vi "COVID_19_CSSE_JHU_Parser.vi"() -> ()   [LabVIEW 2015]
panel:
  out "Graph 2":cluster{"Array out":dbl[], "Array out":dbl[]}[](graph)
  out "Graph":cluster{"Array out":dbl[], dbl[]}[](graph)
  out "Preview":dbl[](graph)
  in  "Population (Millions)":u64 format="%.3p"
  in  "Adjusted by Population (Million)":bool
  in  "Align to First Cases Reported":bool
  in  "State/Province":string(combo)="All"
  in  "Country":string(combo)="All"
  in  "Dataset":enum32{"Confirmed Cases", "Deaths"}(radio)
  in  "Path":path
  in  "reset":bool
  in  "plot":bool
  in  "stop":bool
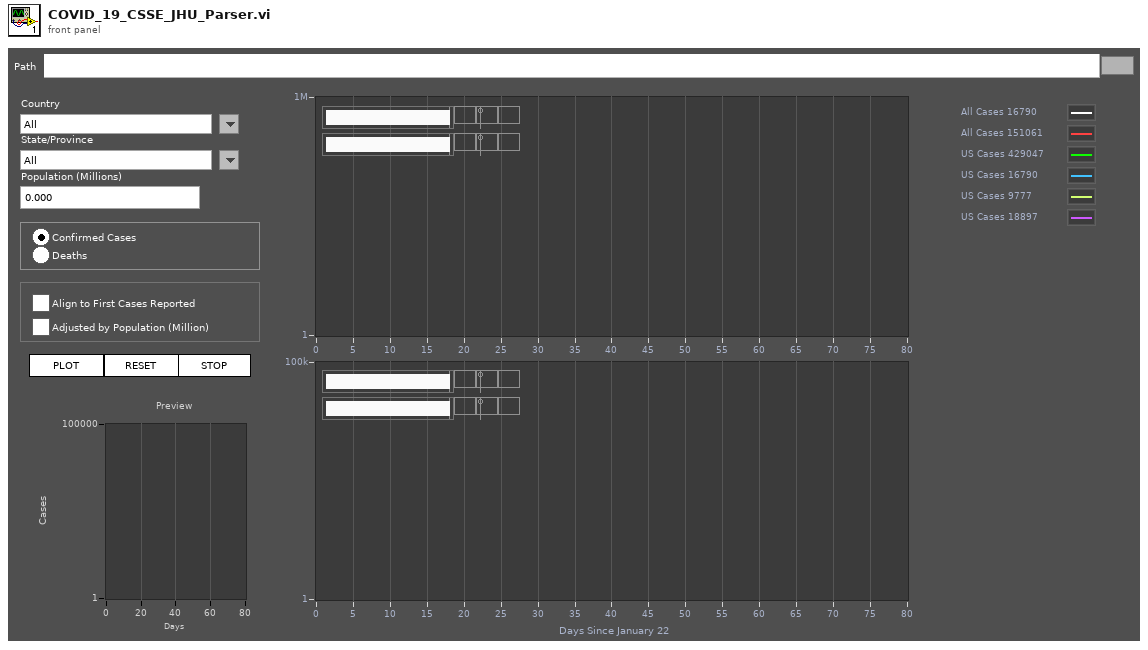
[diagram p1: front panel]
types:
  T1 = enum16{"Initialize", "Start", "Plot", "Reset", "Convert_Data"}
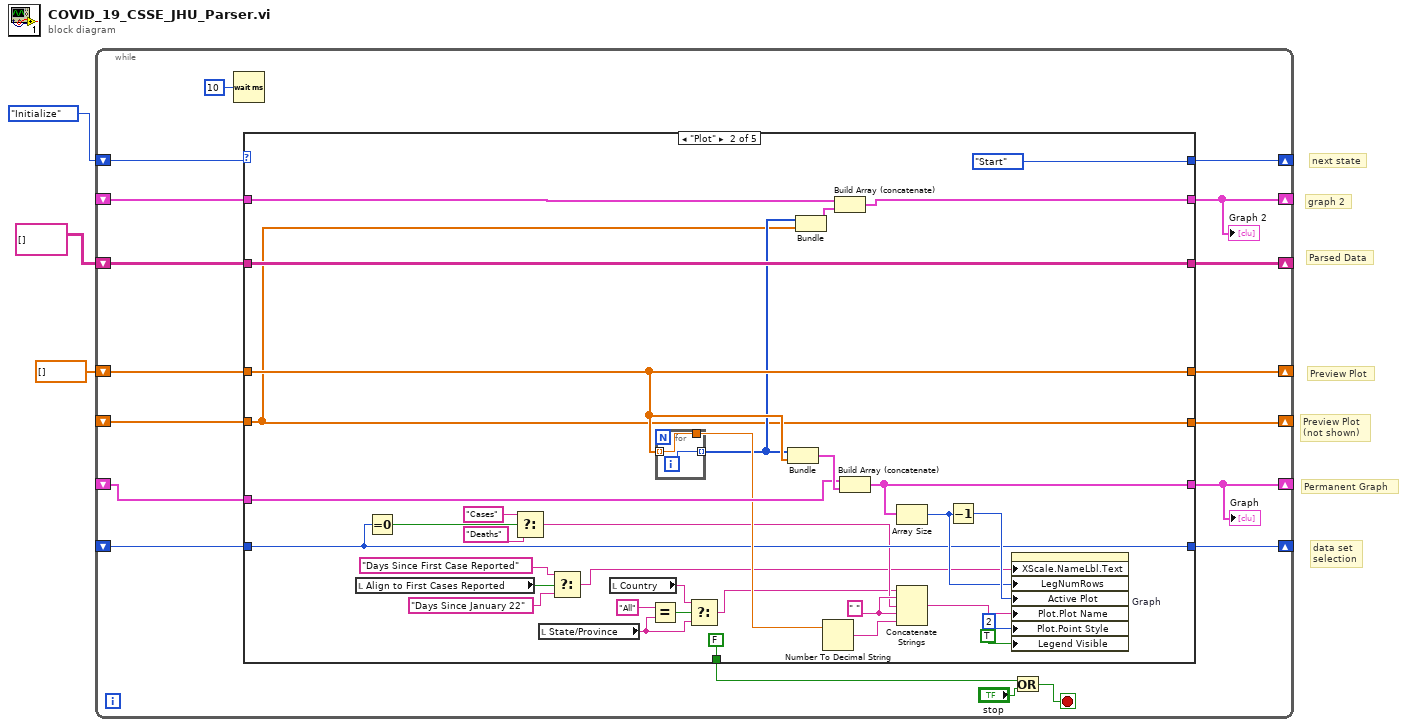
[diagram p0: block diagram]
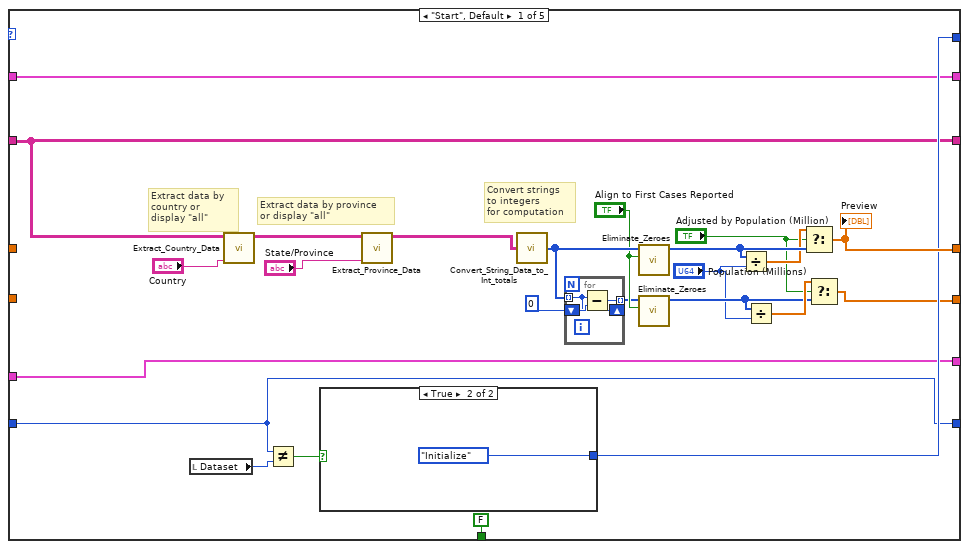
[diagram p2: hidden frame]
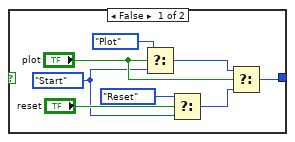
[diagram p3: hidden frame]
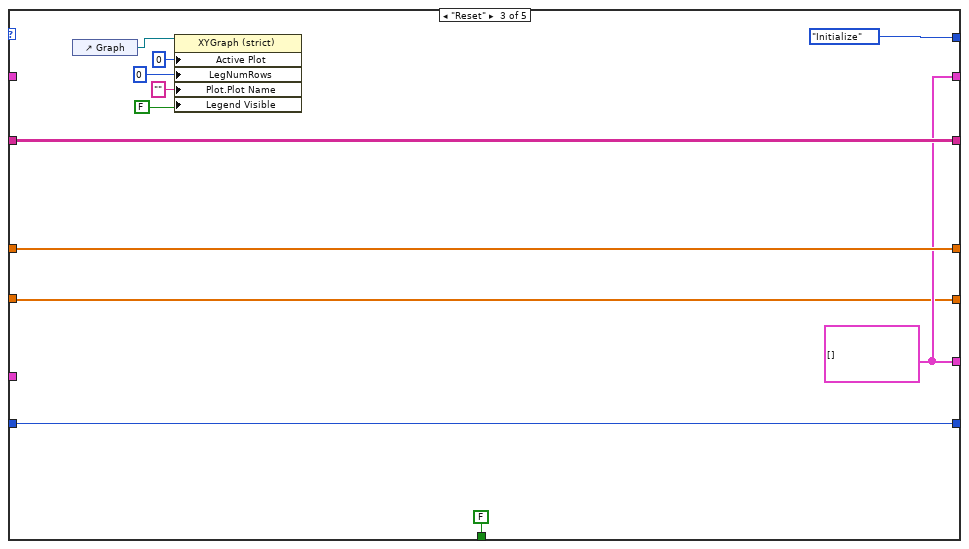
[diagram p4: hidden frame]
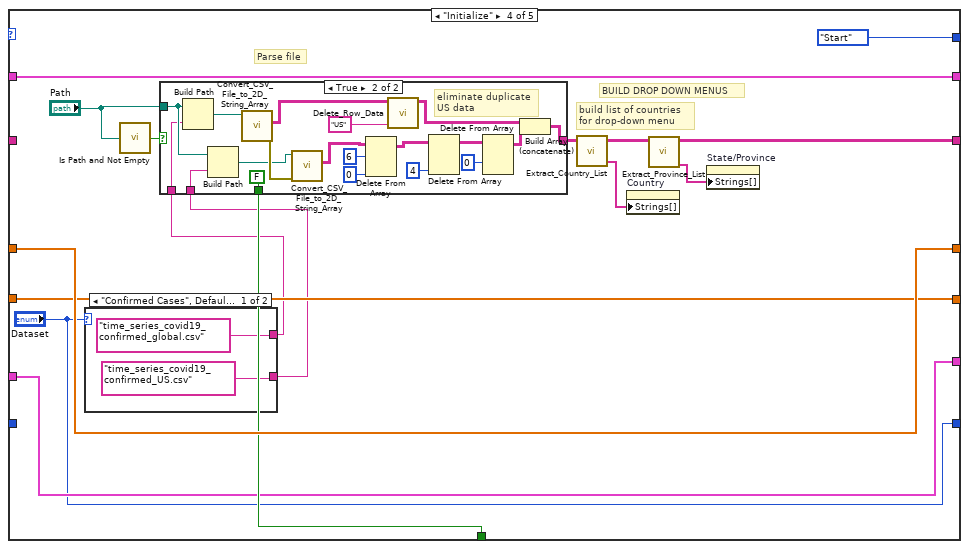
[diagram p5: hidden frame]
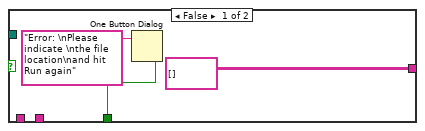
[diagram p6: hidden frame]
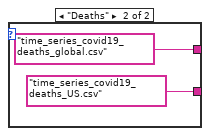
[diagram p7: hidden frame]
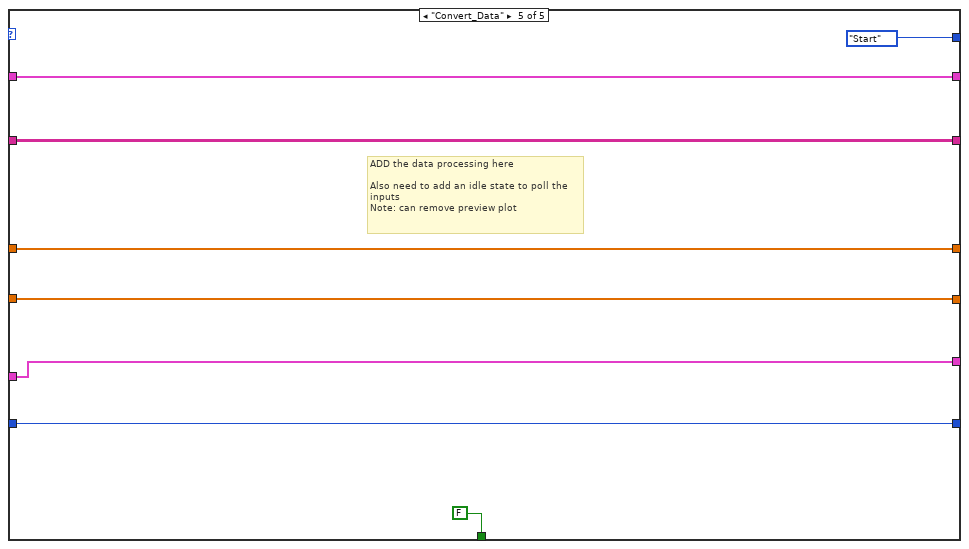
[diagram p8: hidden frame]
diagram:
  # "data set\nselection"
  # "next state"
  # "graph 2"
  # "Preview Plot \n(not shown)"
  # "Parsed Data"
  # "Preview Plot"
  # "Permanent Graph"
  n1 = while {
    shift-right: [w16] -> _
    shift-left: T1."Initialize" -> [w4]
    shift-right: [w20] -> _
    shift-left: string[][] [] ("all rows") -> [w19]
    shift-right: [w18] -> _
    shift-left: dbl[] [] ("Array out") -> [w17]
    shift-right: [w15] -> _
    shift-left: _ -> [w14]
    shift-right: [w13] -> _
    shift-left: _ -> [w12]
    shift-right: [w11] -> _
    shift-left: _ -> [w10]
    shift-right: [w8] -> _
    shift-left: _ -> [w9]
    stop <- w6 stop-if-true
    n2 = Wait (ms)(milliseconds to wait=u32 10) -> ()  [unwired: 1 out]
    n3 = case shown="\"Plot\"" w4 {
      tunnel: [w23 w91 w104 w108 w154] -> w20
      tunnel: w19 -> [w23 w91 w104 _ w154]
      tunnel: [w41 w87 w105 w121 w153] -> w18
      tunnel: w17 -> [_ w87 w105 w121 w153]
      tunnel: [w38 enum16{"Initialize", "Start", "Plot", "Reset"}."Start" enum16{"Initialize", "Start", "Plot", "Reset"}."Initialize" enum16{"Initialize", "Start", "Plot", "Reset"}."Start" T1."Start"] -> w16
      tunnel: [w37 w78 w102 "Dataset" w150] -> w15
      tunnel: w14 -> [w37 w78 w102 _ w150]
      tunnel: [w30 w86 w96 w114 w151] -> w13
      tunnel: w12 -> [w30 w88 _ w114 w151]
      tunnel: [w24 w64 w95 w119 w152] -> w11
      tunnel: w10 -> [_ w64 w95 w119 w152]
      tunnel: [w33 w66 w96 w118 w155] -> w8
      tunnel: w9 -> [w33 w65 _ w118 w155]
      tunnel: [FALSE ("true") FALSE ("true") FALSE ("true") w115 FALSE ("true")] -> w5
      frame "Start", Default {
        # "Extract data by province \nor display \"all\""
        # "Convert strings \nto integers\nfor computation"
        # "Extract data by country or display \"all\""
        n4 = local read "Dataset"() -> (w40:enum32{"Confirmed Cases", "Deaths"})
        n5 = call "Extract_Country_Data.vi"("Country"="Country", "Raw Data Array (String)"=w23) -> ("Country Data"=w22:string[][])  [unwired: 9 in]
        n6 = Not Equal?(x=w37, y=w40) -> (x != y?=w39:bool)
        n7 = case shown="True" w39 {
          tunnel: [w54 enum16{"Initialize", "Start", "Plot", "Reset"}."Initialize"] -> w38
          frame False {
            w50 = enum16{"Initialize", "Start", "Plot", "Reset"}."Start"
            n8 = Select(t=enum16{"Initialize", "Start", "Plot", "Reset"}."Plot", s="plot", f=w50) -> (s? t:f=w53:enum16{"Initialize", "Start", "Plot", "Reset"})
            n9 = Select(t=enum16{"Initialize", "Start", "Plot", "Reset"}."Reset", s="reset", f=w50) -> (s? t:f=w49:enum16{"Initialize", "Start", "Plot", "Reset"})
            n10 = Select(t=w53, s="plot", f=w49) -> (s? t:f=w54:enum16{"Initialize", "Start", "Plot", "Reset"})
          }
          frame True {
          }
        }
        n11 = call "Extract_Province_Data.vi"("Province"="State/Province", "Country Data In"=w22) -> ("Province Data Out"=w43:string[][])  [unwired: 9 in]
        n12 = call "Convert_String_Data_to_Int_totals.vi"("Province Data Out"=w43) -> ("Array"=w36:i32[])
        n13 = for {
          tunnel: w36 -> [w46] mode=indexing
          shift-right: [w46] -> _
          shift-left: 0 -> [w48]
          tunnel: [w47] -> w31 mode=indexing
          n14 = Subtract(x=w46, y=w48) -> (x-y=w47:i32)
        }
        n15 = call "Eliminate_Zeroes.vi"("Align to First Cases Reported"="Align to First Cases Reported", "Array in"=w36) -> ("Array out"=w42:i32[])  [unwired: 9 in]
        n16 = call "Eliminate_Zeroes.vi"("Align to First Cases Reported"="Align to First Cases Reported", "Array in"=w31) -> ("Array out"=w27:i32[])  [unwired: 9 in]
        n17 = Divide(x=w42, y="Population (Millions)") -> (x/y=w29:dbl[])
        n18 = Divide(x=w27, y="Population (Millions)") -> (x/y=w28:dbl[])
        n19 = Select(t=w29, s="Adjusted by Population (Million)", f=w42) -> (s? t:f=w41:dbl[])
        "Preview" <- w41
        n20 = Select(t=w28, s="Adjusted by Population (Million)", f=w27) -> (s? t:f=w24:dbl[])
      }
      frame "Plot" {
        w74 = " " ("string")
        n21 = local read "Align to First Cases Reported"() -> (w70:bool)
        n22 = Equal To 0?(x=w78) -> (x = 0?=w77:bool)
        n23 = Select(t="Cases" ("string"), s=w77, f="Deaths" ("string")) -> (s? t:f=w73:string)
        n24 = local read "State/Province"() -> (w59:string)
        n25 = Select(t="Days Since First Case Reported" ("string"), s=w70, f="Days Since January 22" ("string")) -> (s? t:f=w69:string)
        n26 = local read "Country"() -> (w60:string)
        n27 = Equal?(x="All", y=w59) -> (x = y?=w61:bool)
        n28 = for {
          tunnel: w87 -> [w93] mode=indexing
          tunnel: [w92] -> w67 mode=indexing
          tunnel: [w93] -> w79
          i -> [w92]
        }
        n29 = Select(t=w60, s=w61, f=w59) -> (s? t:f=w58:string)
        n30 = Bundle(w67, "Array out"=w87) -> (w89:cluster{i32[], "Array out":dbl[]})  [unwired: 1 in]
        n31 = Bundle(w67, "Array out"=w64) -> (w68:cluster{i32[], "Array out":dbl[]})  [unwired: 1 in]
        n32 = Number To Decimal String(number=w79) -> (decimal integer string=w80:string)  [unwired: 1 in]
        n33 = Build Array (concatenate)(w65, w68) -> (w66:cluster{"Array out":dbl[], "Array out":dbl[]}[])
        n34 = Build Array (concatenate)(w88, w89) -> (w86:cluster{"Array out":dbl[], "Array out":dbl[]}[])
        n35 = Array Size(array=w86) -> (size(s)=w84:i32)
        n36 = Concatenate Strings(w58, w74, w73, w74, w80) -> (w81:string)
        n37 = Decrement(x=w84) -> (x-1=w85:i32)
        n38 = property on="Graph" class="XYGraph (strict)"("XScale.NameLbl.Text"=w69, "LegNumRows"=w84, "Active Plot"=w85, "Plot.Plot Name"=w81, "Plot.Point Style"=u8 2, "Legend Visible"=TRUE ("Legend:Visible")) -> ()  [unwired: 2 in, 2 out]
      }
      frame "Reset" {
        w96 = cluster{"Array out":dbl[], dbl[]}[] []
        n39 = control-ref of="Graph"() -> (w100:refnum<vi>)
        n40 = property on="Property Node" class="XYGraph (strict)"(reference=w100, "Active Plot"=u32 0, "LegNumRows"=u32 0 ("Legend:Number of Rows"), "Plot.Plot Name"="", "Legend Visible"=FALSE ("Legend:Visible")) -> ()  [unwired: 1 in, 2 out]
      }
      frame "Initialize" {
        # "BUILD DROP DOWN MENUS"
        # "build list of countries\nfor drop-down menu"
        # "Parse file"
        n41 = case shown="\"Confirmed Cases\", Default" "Dataset" {
          tunnel: ["time_series_covid19_confirmed_global.csv" "time_series_covid19_deaths_global.csv"] -> w111
          tunnel: ["time_series_covid19_confirmed_US.csv" "time_series_covid19_deaths_US.csv"] -> w110
          frame "Confirmed Cases", Default {
          }
          frame "Deaths" {
          }
        }
        n42 = call <vilib>:"Is Path and Not Empty.vi"("path"="Path") -> ("Is Path and Not Empty?"=w117:bool)  [unwired: 4 in]
        n43 = case shown="True" w117 {
          tunnel: [string[][] [] ("all rows") w133] -> w112
          tunnel: "Path" -> [_ w141]
          tunnel: [w122 FALSE ("true")] -> w115
          tunnel: w111 -> [_ w126]
          tunnel: w110 -> [_ w125]
          frame False {
            n44 = One Button Dialog(message="Error: \nPlease indicate \nthe file location\nand hit Run again") -> (true=w122:bool)  [unwired: 1 in]
          }
          frame True {
            # "eliminate duplicate\nUS data"
            n45 = Build Path(base path=w141, name or relative path=w126) -> (appended path=w142:path)
            n46 = Build Path(base path=w141, name or relative path=w125) -> (appended path=w139:path)
            n47 = call "Convert_CSV_File_to_2D_String_Array.vi"("CSV File Path"=w142) -> ("error out"=w140:errorcluster, "2-D Array"=w129:string[][])  [unwired: 8 in, 1 out]
            n48 = call "Convert_CSV_File_to_2D_String_Array.vi"("error in"=w140, "CSV File Path"=w139) -> ("2-D Array"=w138:string[][])  [unwired: 7 in, 2 out]
            n49 = Delete From Array(array=w138, length=6, index (col)=0 ("disabled index (col)")) -> (array with subset deleted=w135:string[][])  [unwired: 1 in, 1 out]
            n50 = call "Delete_Row_Data.vi"("Country"="US", "Raw Data Array (String)"=w129) -> ("array w/ subset deleted"=w127:string[][])  [unwired: 9 in]
            n51 = Delete From Array(array=w135, index (col)=4 ("disabled index (col)")) -> (array with subset deleted=w132:string[][])  [unwired: 2 in, 1 out]
            n52 = Delete From Array(array=w132, index (row)=0) -> (array with subset deleted=w130:string[][])  [unwired: 2 in, 1 out]
            n53 = Build Array (concatenate)(w127, w130) -> (w133:string[][])
          }
        }
        n54 = call "Extract_Country_List.vi"("Raw Data Array (String)"=w112) -> ("List of Countries"=w106:string[], "Raw Data Array Out (String)"=w109:string[][])  [unwired: 3 in]
        n55 = property on="Country" class="CmbBox"("Strings[]"=w106) -> ()  [unwired: 2 in, 2 out]
        n56 = call "Extract_Province_List.vi"("Country Data In"=w109) -> ("Province List"=w107:string[], "Country Data Out"=w108:string[][])  [unwired: 9 in]
        n57 = property on="State/Province" class="CmbBox"("Strings[]"=w107) -> ()  [unwired: 2 in, 2 out]
      }
      frame "Convert_Data" {
        # "ADD the data processing here\n\nAlso need to add an idle state to poll the inputs\nNote: can remove preview plot"
      }
    }
    "Graph" <- w13
    "Graph 2" <- w8
    n58 = Or(x=w5, y="stop") -> (x .or. y?=w6:bool)
  }
